vi "IsChanged.vi"(3 "Reset":bool caption="Reset (F)", 4 "Data":variant) -> (1 "Data Changed?":bool)   [LabVIEW 2017, in "GPComparison.lvlib"]
doc: "Wire anything to <B>Data</B> and <B>Data Changed?</B> will be True if data differs from the last data that was input.\n\n<B>Data Changed?</B> will always be False on first call and when <B>Reset</B> is True.\n\nThis VI is inlined.\n\nSteen Schmidt\nGPower\n22/10 2016"
uses:
  GPComparison.lvlib
panel:
  # "Copyright © 2016\nGPower\nSee enclosed license file for terms and conditions"
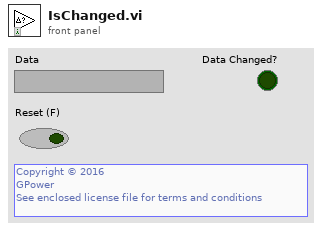
[diagram p1: front panel]
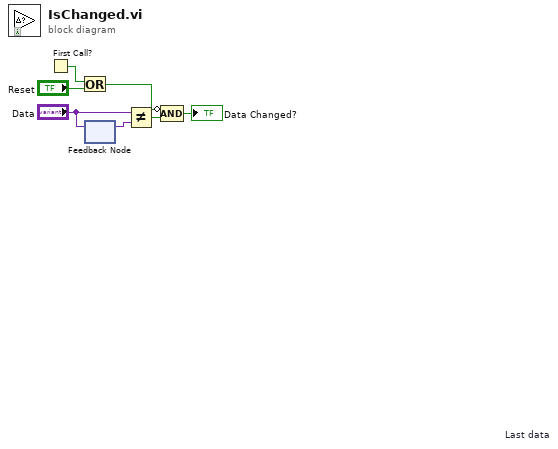
[diagram p0: block diagram]
diagram:
  n1 = First Call?() -> (First Call?: T/F=w3:bool)
  n2 = Or(x=w3, y="Reset") -> (x .or. y?=w1:bool)
  n3 = feedback-in #1("Data") -> ()
  n4 = feedback #1 "Last data"() -> (w7:variant)  [unwired: 1 in]
  n5 = Not Equal?(x="Data", y=w7) -> (x != y?=w6:bool)
  n6 = Compound Arithmetic op=AND(invert w1, w6) -> (→"Data Changed?":bool)
